vi "PLC Struct Byte Stream to Data String.vi"(8 "error in (no error)":errorcluster, 9 "[Sub-Item Type Information]":T1[](array[typedef]), 10 "Byte Stream":u8[](array[numeric]), 11 "TwinCAT ADS in":refnum<class "TwinCAT ADS.lvclass">) -> (0 "error out":errorcluster, 1 "Data String":string, 2 "Type Descriptor":i16[](array[numeric]), 3 "TwinCAT ADS out":refnum<class "TwinCAT ADS.lvclass">)   [LabVIEW 2018, in "TwinCAT ADS.lvclass"]
uses:
  TwinCAT ADS.lvclass
  Controls/PLC Sub-Item Type Descriptor.ctl
  Controls/PLC Type.ctl
  PLC Primitive Byte Stream to Data String.vi/dd5e40b3-f89d-44d0-b911-1f2dc1f1e391.vi
  PLC Primitive Byte Stream to Data String.vi/9a8c356b-cf55-4838-9201-0532b80217b2.vi
  PLC Primitive Byte Stream to Data String.vi/06482052-d1f9-4f29-aca9-908031c6a69f.vi
  PLC Primitive Byte Stream to Data String.vi/b9242781-96b0-446e-9150-452b1084ed54.vi
  PLC Primitive Byte Stream to Data String.vi/5fbe6976-0b86-40a2-b7b6-3748894f0071.vi
  PLC Primitive Byte Stream to Data String.vi/c4de1741-fffd-4fed-ba25-d7b4acbf0555.vi
  PLC Primitive Byte Stream to Data String.vi/20356124-05d2-4a04-a5d1-e69adc4c58c2.vi
  PLC Primitive Byte Stream to Data String.vi/67ddb754-0fbe-43d9-9e61-34d6659124ef.vi
  PLC Primitive Byte Stream to Data String.vi/e3d41cb3-d20e-45e9-8252-e41884a8f4d0.vi
  PLC Primitive Byte Stream to Data String.vi/46ba2a54-cc07-4222-9a0e-bd972edfcef0.vi
  PLC Primitive Byte Stream to Data String.vi/6b416cf7-30dc-48a3-9278-9d800f443678.vi
  PLC Primitive Byte Stream to Data String.vi/5857d013-9824-4299-a2d7-53efdc0d26c5.vi
  PLC Primitive Byte Stream to Data String.vi/006b0e7e-7e80-41f3-be4e-1f3da8479fae.vi
  PLC Primitive Byte Stream to Data String.vi/28d9c90b-5f2a-4c58-95e2-5fc46303b0fd.vi
  PLC Primitive Byte Stream to Data String.vi/99b7bc4a-962e-4818-aa5d-444f23f83b11.vi
  PLC Primitive Byte Stream to Data String.vi/8b7c42c8-9170-4542-8f35-15cbeddc22cb.vi
  PLC Primitive Byte Stream to Data String.vi/65a091fa-0bd2-4a35-ae2b-3fa5e90d1994.vi
  PLC Primitive Byte Stream to Data String.vi/4b7d3a7d-7f1b-46f0-9357-48cb72148c56.vi
  PLC Primitive Byte Stream to Data String.vi/b431183c-2ad5-4c6d-9bfa-a53b18913682.vi
  PLC Primitive Byte Stream to Data String.vi/30c6c28a-53c3-4e33-80b1-b22f521e1f67.vi
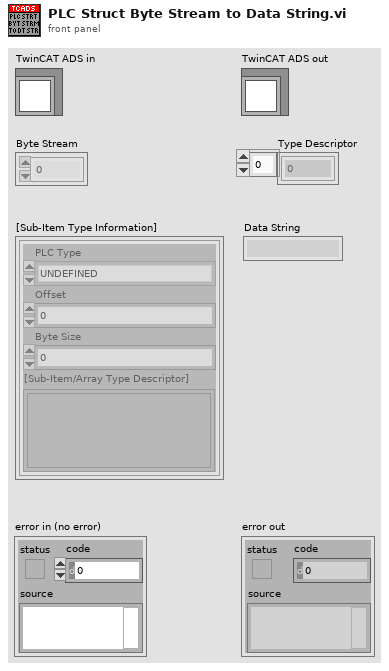
[diagram p1: front panel]
types:
  T1 = typedef "TwinCAT ADS.lvclass/PLC Sub-Item Type Descriptor.ctl" = cluster{"PLC Type":T2, "Offset":i32, "Byte Size":i32, "[Sub-Item/Array Type Descriptor]":variant[]}
  T2 = typedef "TwinCAT ADS.lvclass/PLC Type.ctl" = enum16{"UNDEFINED", "INT", "DINT", "REAL", "LREAL", "SINT", "BYTE", "UINT", "UDINT", "LINT", "ULINT", "STRING", "WSTRING", "BOOL", "TIME", "LTIME", "DATE", "DT", "TOD", "ARRAY", "JAGGED ARRAY", "STRUCT", "FUNCTION BLOCK", "UNION", "POINTER", "USER DEFINED"}
  T3 = typedef "TwinCAT ADS.lvclass/PLC Array Type Descriptor.ctl" = cluster{"Fundamental PLC Type":T2, "Fundamental Type Byte Size":i32, "Item Count":i32, "Dimension Lengths":i32[], "Sub-Item Type Descriptor":variant}
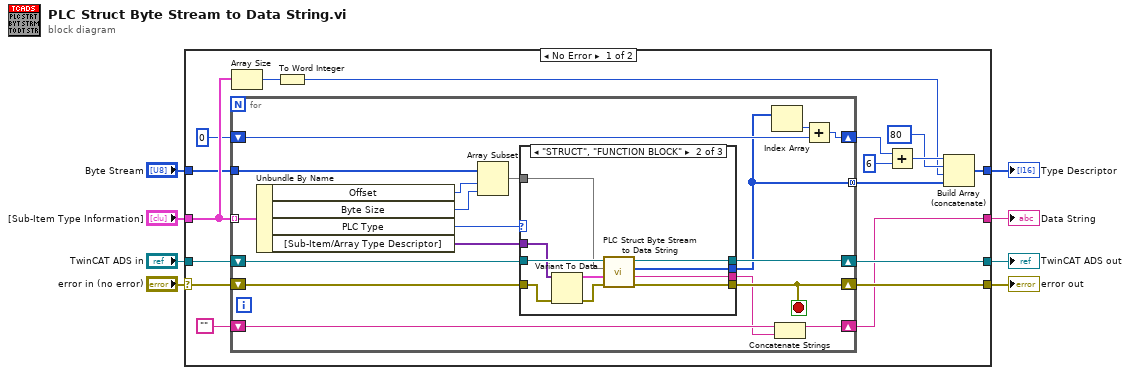
[diagram p0: block diagram]
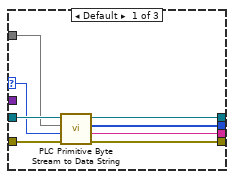
[diagram p2: hidden frame]
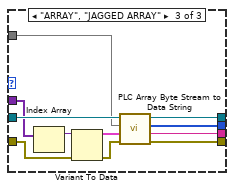
[diagram p3: hidden frame]
diagram:
  n1 = case shown="No Error" "error in (no error)" {
    selector: "error in (no error)" -> [w14 w74]
    tunnel: "[Sub-Item Type Information]" -> [w25 _]
    tunnel: "TwinCAT ADS in" -> [w24 w73]
    tunnel: "Byte Stream" -> [w23 _]
    tunnel: [w17 w73] -> w5
    tunnel: [w10 w74] -> w4
    tunnel: [w11 _] -> w2
    tunnel: [w9 _] -> w1
    frame No Error {
      n2 = for {
        shift-right: [w39] -> w17
        shift-left: w24 -> [w43]
        tunnel: w25 -> [w38] mode=indexing
        shift-right: [w30] -> w10
        shift-left: w14 -> [w42]
        shift-right: [w36] -> w16
        shift-left: i16 0 -> [w35]
        tunnel: w23 -> [w34]
        shift-right: [w28] -> w9
        shift-left: "" -> [w29]
        tunnel: [w27] -> w15 mode=concatenating
        stop <- w30 stop-if-true
        n3 = Unbundle By Name(w38) -> ("Offset"=w33:i32, "Byte Size"=w32:i32, "PLC Type"=w41:T2, "[Sub-Item/Array Type Descriptor]"=w40:variant[])
        n4 = Array Subset(array=w34, index=w33, length=w32) -> (w31:u8[])
        n5 = case shown="\"STRUCT\", \"FUNCTION BLOCK\"" w41 {
          selector: w41 -> [w45 _ _]
          tunnel: w43 -> [w51 w61 w72]
          tunnel: w42 -> [w50 w57 w70]
          tunnel: w31 -> [w44 w60 w66]
          tunnel: [w49 w59 w65] -> w39
          tunnel: [w48 w58 w64] -> w30
          tunnel: w40 -> [_ w56 w71]
          tunnel: [w47 w52 w63] -> w27
          tunnel: [w46 w53 w62] -> w26
          frame Default {
            n6 = call "PLC Primitive Byte Stream to Data String.vi"("error in (no error)"=w50, "PLC Type"=w45, "Byte Stream"=w44, "TwinCAT ADS in"=w51) -> ("error out"=w48:errorcluster, "Data String"=w46:string, "Type Descriptor"=w47:i16[], "TwinCAT ADS out"=w49:refnum<class "TwinCAT ADS.lvclass">)  [unwired: 4 in]
          }
          frame "STRUCT", "FUNCTION BLOCK" {
            n7 = Variant To Data(error in=w57, Variant=w56) -> (data=w54:T1[], error out=w55:errorcluster)  [unwired: 1 in]
            n8 = call "PLC Struct Byte Stream to Data String.vi"("error in (no error)"=w55, "[Sub-Item Type Information]"=w54, "Byte Stream"=w60, "TwinCAT ADS in"=w61) -> ("error out"=w58:errorcluster, "Data String"=w53:string, "Type Descriptor"=w52:i16[], "TwinCAT ADS out"=w59:refnum<class "TwinCAT ADS.lvclass">)  [unwired: 4 in]
          }
          frame "ARRAY", "JAGGED ARRAY" {
            n9 = Index Array(array=w71) -> (element=w69:variant)  [unwired: 1 in]
            n10 = Variant To Data(error in=w70, Variant=w69) -> (data=w68:T3, error out=w67:errorcluster)  [unwired: 1 in]
            n11 = call "PLC Array Byte Stream to Data String.vi"("error in (no error)"=w67, "Array Type Descriptor"=w68, "Byte Stream"=w66, "TwinCAT ADS in"=w72) -> ("error out"=w64:errorcluster, "Data String"=w62:string, "Type Descriptor"=w63:i16[], "TwinCAT ADS out"=w65:refnum<class "TwinCAT ADS.lvclass">)  [unwired: 4 in]
          }
        }
        n12 = Index Array(array=w27) -> (element=w37:i16)  [unwired: 1 in]
        n13 = Concatenate Strings(w29, w26) -> (w28:string)
        n14 = Add(x=w37, y=w35) -> (x+y=w36:i16)
      }
      n15 = Array Size(array=w25) -> (size(s)=w22:i32)
      n16 = To Word Integer(number=w22) -> (16bit integer=w18:i16)
      n17 = Add(x=w16, y=i16 6) -> (x+y=w20:i16)
      n18 = Build Array (concatenate)(w20, i16 80, w18, w15) -> (w11:i16[])
    }
    frame Error {
    }
  }
  "error out" <- w4
  "TwinCAT ADS out" <- w5
  "Data String" <- w1
  "Type Descriptor" <- w2
